vi "12 - Data-source attach.vi"() -> ()   [LabVIEW 2020]
uses:
  client/client.lvlib
panel:
  out "Source Type":i32
  out "Source Name":string
  out "Source Count":u32
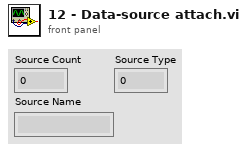
[diagram p1: front panel]
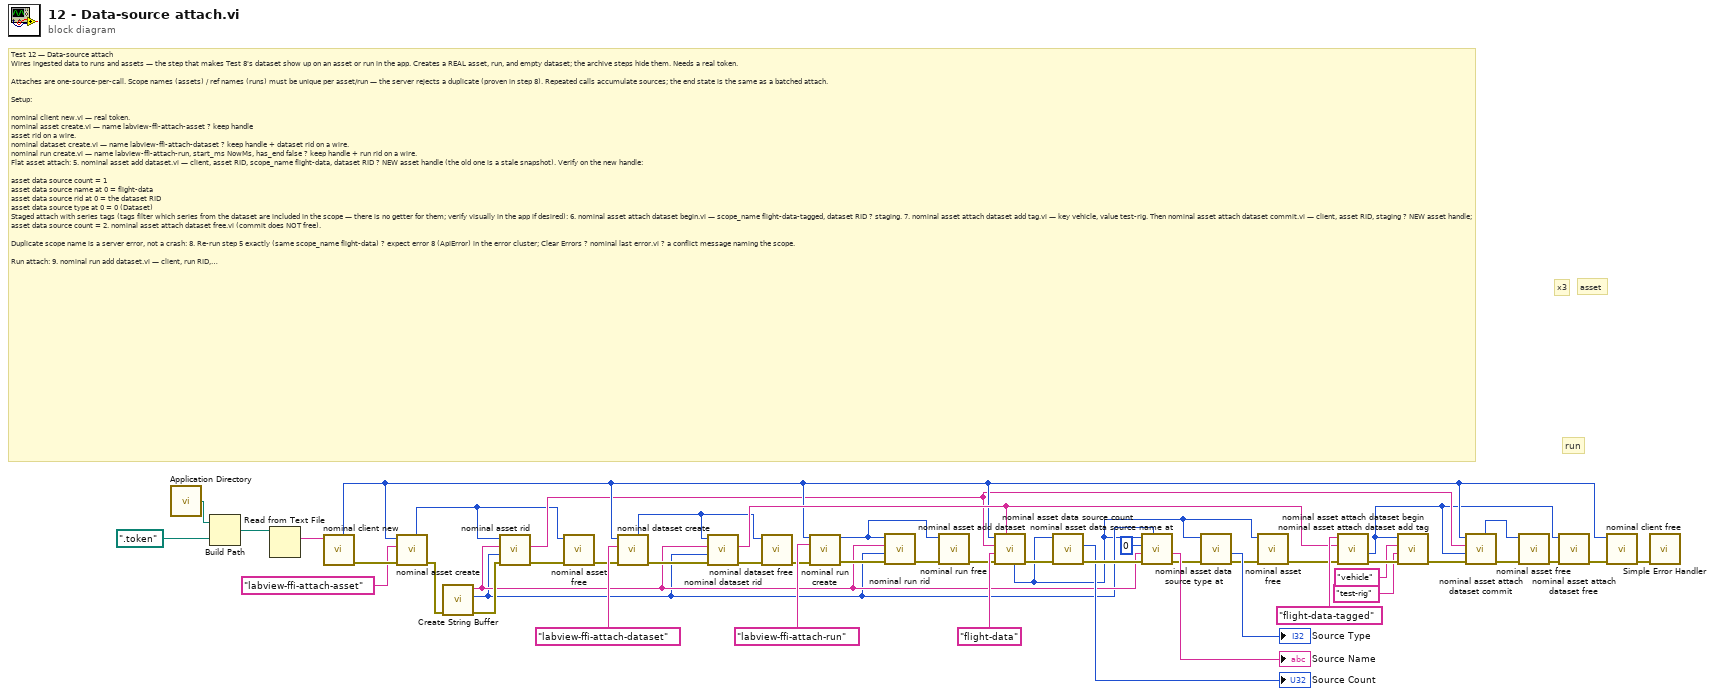
[diagram p0: block diagram]
diagram:
  # "run"
  # "asset"
  # "x3"
  # "Test 12 — Data-source attach\nWires ingested data to runs and assets — the step that makes Test 8's dataset show up on an asset or run in the app. Creates a REAL asset, run, and empty dataset; the archive steps hide them. Needs a real token.\n\nAttaches are one-source-per-call. Scope names (assets) / ref names (runs) must be unique per asset/run — the server rejects a duplicate (proven in step 8). Repeated calls accumulate sources; the end state is the same as a batched attach.\n\nSetup:\n\nnominal client new.vi — real token.\nnominal asset create.vi — name labview-ffi-attach-asset ? keep handle\nasset rid on a wire.\nnominal dataset create.vi — name labview-ffi-attach-dataset ? keep handle + dataset rid on a wire.\nnominal run create.vi — name labview-ffi-attach-run, start_ms NowMs, has_end false ? keep handle + run rid on a wire.\nFlat asset attach: 5. nominal asset add dataset.vi — client, asset RID, scope_name flight-data, dataset RID ? NEW asset handle (the old one is a stale snapshot). Verify on the new handle:\n\nasset data source count = 1\nasset data source name at 0 = flight-data\nasset data source rid at 0 = the dataset RID\nasset data source type at 0 = 0 (Dataset)\nStaged attach with series tags (tags filter which series from the dataset are included in the scope — there is no getter for them; verify visually in the app if desired): 6. nominal asset attach dataset begin.vi — scope_name flight-data-tagged, dataset RID ? staging. 7. nominal asset attach dataset add tag.vi — key vehicle, value test-rig. Then nominal asset attach dataset commit.vi — client, asset RID, staging ? NEW asset handle; asset data source count = 2. nominal asset attach dataset free.vi (commit does NOT free).\n\nDuplicate scope name is a server error, not a crash: 8. Re-run step 5 exactly (same scope_name flight-data) ? expect error 8 (ApiError) in the error cluster; Clear Errors ? nominal last error.vi ? a conflict message naming the scope.\n\nRun attach: 9. nominal run add dataset.vi — client, run RID, ref_name flight-data, dataset RID ? NEW run handle. Verify: run data source count = 1, run data source name at 0 = flight-data, run data source rid at 0 = the dataset RID, run data source type at 0 = 0. (nominal asset add video.vi / add connection.vi and the run equivalents are the same shape — covered by the automated suite; spot check them here only if you have a real video/connection RID handy.)\n\nCleanup: 10. nominal run archive.vi, nominal asset archive.vi, nominal dataset archive.vi — client + each RID. 11. Free every handle: both extra asset handles from steps 5/7, the run handle from step 9, the originals from setup, then nominal client free.vi."
  n1 = call <vilib>:"Application Directory.vi"() -> ("Application Directory"=w47:path)
  n2 = Build Path(base path=w47, name or relative path=path ".token") -> (appended path=w45:path)
  n3 = Read from Text File(file (use dialog)=w45) -> (text=w44:string)  [unwired: 3 in, 3 out]
  n4 = call "nominal client new.vi"("token"=w44) -> ("error out"=w43:errorcluster, "out_client out"=w20:i32)  [unwired: 8 in, 1 out]
  n5 = call "nominal asset create.vi"("error in (no error)"=w43, "name"="labview-ffi-attach-asset", "client"=w20) -> ("error out"=w40:errorcluster, "out_asset out"=w6:i32)  [unwired: 6 in, 1 out]
  n6 = call "Create String Buffer.vi"("error in"=w40) -> ("error out"=w39:errorcluster, "dub Buffer Size"=w28:i32, "String Buffer"=w30:string)  [unwired: 8 in]
  n7 = call "nominal asset rid.vi"("error in (no error)"=w39, "cap"=w28, "buf"=w30, "asset"=w6) -> ("error out"=w5:errorcluster, "buf out"=w19:string)  [unwired: 4 in, 2 out]
  n8 = call "nominal asset free.vi"("error in (no error)"=w5, "asset"=w6) -> ("error out"=w4:errorcluster)  [unwired: 8 in, 1 out]
  n9 = call "nominal dataset create.vi"("error in (no error)"=w4, "name"="labview-ffi-attach-dataset", "client"=w20) -> ("error out"=w32:errorcluster, "out_dataset out"=w12:i32)  [unwired: 6 in, 1 out]
  n10 = call "nominal dataset rid.vi"("error in (no error)"=w32, "cap"=w28, "buf"=w30, "dataset"=w12) -> ("error out"=w11:errorcluster, "buf out"=w24:string)  [unwired: 4 in, 2 out]
  n11 = call "nominal dataset free.vi"("error in (no error)"=w11, "dataset"=w12) -> ("error out"=w10:errorcluster)  [unwired: 8 in, 1 out]
  n12 = call "nominal run create.vi"("client"=w20, "name"="labview-ffi-attach-run", "error in (no error)"=w10) -> ("out_run out"=w9:i32, "error out"=w33:errorcluster)  [unwired: 10 in, 1 out]
  n13 = call "nominal run rid.vi"("error in (no error)"=w33, "cap"=w28, "buf"=w30, "run"=w9) -> ("error out"=w8:errorcluster)  [unwired: 4 in, 3 out]
  n14 = call "nominal run free.vi"("error in (no error)"=w8, "run"=w9) -> ("error out"=w7:errorcluster)  [unwired: 8 in, 1 out]
  n15 = call "nominal asset add dataset.vi"("dataset_rid"=w24, "error in (no error)"=w7, "scope_name"="flight-data" ("name"), "rid"=w19, "client"=w20) -> ("error out"=w36:errorcluster, "out_asset out"=w15:i32)  [unwired: 4 in, 1 out]
  n16 = call "nominal asset data source count.vi"("error in (no error)"=w36, "asset"=w15) -> ("error out"=w34:errorcluster, "out_count out"=→"Source Count":u32)  [unwired: 7 in, 1 out]
  n17 = call "nominal asset data source name at.vi"("cap"=w28, "error in (no error)"=w34, "buf"=w30, "index"=0, "asset"=w15) -> ("error out"=w27:errorcluster, "buf out"=→"Source Name":string)  [unwired: 3 in, 2 out]
  n18 = call "nominal asset data source type at.vi"("error in (no error)"=w27, "asset"=w15) -> ("error out"=w14:errorcluster, "out_type out"=→"Source Type":i32)  [unwired: 7 in, 1 out]
  n19 = call "nominal asset free.vi"("error in (no error)"=w14, "asset"=w15) -> ("error out"=w13:errorcluster)  [unwired: 8 in, 1 out]
  n20 = call "nominal asset attach dataset begin.vi"("error in (no error)"=w13, "dataset_rid"=w24, "scope_name"="flight-data-tagged") -> ("error out"=w23:errorcluster, "out_staging out"=w17:i32)  [unwired: 6 in, 1 out]
  n21 = call "nominal asset attach dataset add tag.vi"("error in (no error)"=w23, "value"="test-rig", "key"="vehicle", "staging"=w17) -> ("error out"=w18:errorcluster)  [unwired: 6 in, 1 out]
  n22 = call "nominal asset attach dataset commit.vi"("error in (no error)"=w18, "staging"=w17, "rid"=w19, "client"=w20) -> ("error out"=w2:errorcluster, "out_asset out"=w3:i32)  [unwired: 5 in, 1 out]
  n23 = call "nominal asset free.vi"("error in (no error)"=w2, "asset"=w3) -> ("error out"=w1:errorcluster)  [unwired: 8 in, 1 out]
  n24 = call "nominal asset attach dataset free.vi"("error in (no error)"=w1, "staging"=w17) -> ("error out"=w16:errorcluster)  [unwired: 8 in, 1 out]
  n25 = call "nominal client free.vi"("error in (no error)"=w16, "client"=w20) -> ("error out"=w48:errorcluster)  [unwired: 8 in, 1 out]
  n26 = call <vilib>:"Simple Error Handler.vi"("error in (no error)"=w48) -> ()  [unwired: 4 in, 5 out]
